vi "Read Manifold Channel Mapping.vi"(8 "error in (no error)":errorcluster, 11 "Gantry in":refnum<class "Gantry.lvclass">) -> (0 "error out":errorcluster, 1 "Port -> Channel":map{i32, i32}(c390), 2 "Channel -> Port":map{i32, i32}(c390), 3 "Gantry out":refnum<class "Gantry.lvclass">)   [LabVIEW 2026, in "Gantry.lvclass"]
uses:
  Gantry.lvclass
  Gantry.lvclass/Gantry.ctl
  FlexWorktable/FlexWorktable.lvclass
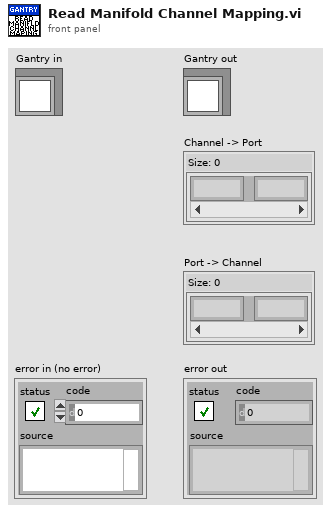
[diagram p1: front panel]
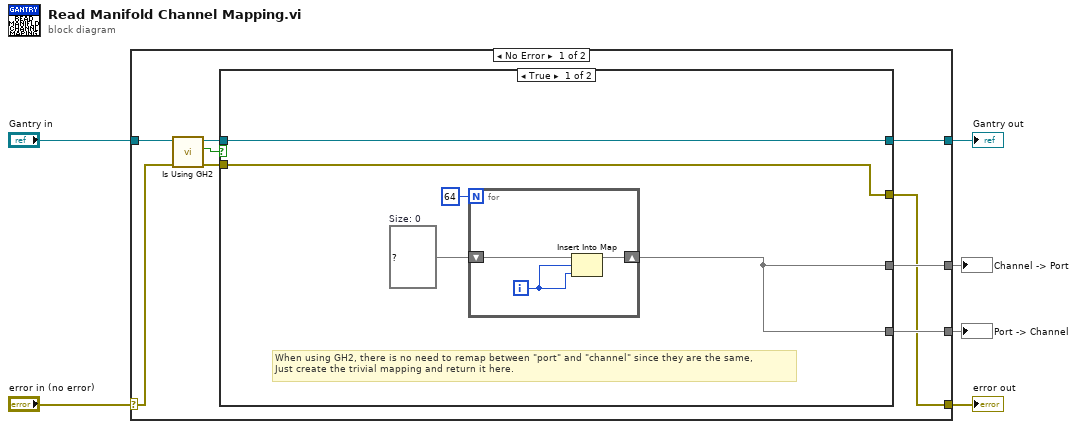
[diagram p0: block diagram]
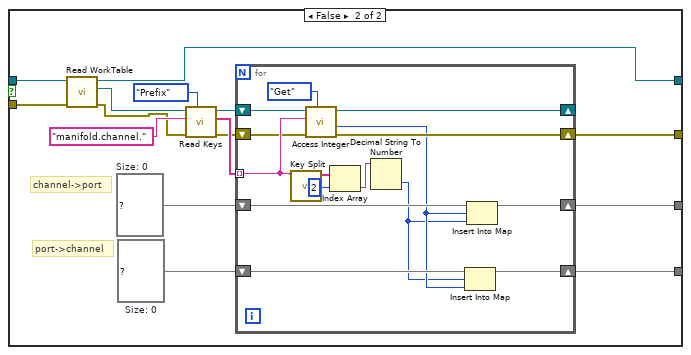
[diagram p2: hidden frame]
diagram:
  n1 = case shown="No Error" "error in (no error)" {
    selector: "error in (no error)" -> [w10 w55]
    tunnel: [w13 w55] -> w5
    tunnel: [w12 w54] -> w3
    tunnel: "Gantry in" -> [w11 w54]
    tunnel: [w15 _] -> w2
    tunnel: [w14 _] -> w1
    frame No Error {
      n2 = call "Is Using GH2.vi"("error in (no error)"=w10, "Gantry in"=w11) -> ("error out"=w9:errorcluster, "Using GH2"=w7:bool, "Gantry out"=w8:refnum<class "Gantry.lvclass">)  [unwired: 7 in]
      n3 = case shown="True" w7 {
        tunnel: w8 -> [w20 w38]
        tunnel: w9 -> [w19 w37]
        tunnel: [w16 w27] -> w15
        tunnel: [w16 w26] -> w14
        tunnel: [w19 w25] -> w13
        tunnel: [w20 w24] -> w12
        frame True {
          w17 = map{i32, i32} {}  # Size: 0
          # "When using GH2, there is no need to remap between \"port\" and \"channel\" since they are the same,\nJust create the trivial mapping and return it here."
          n4 = for {
            N: 64 -> [_]
            shift-right: [w22] -> w16
            shift-left: w17 -> [w23]
            i -> [w21]
            n5 = Insert Into Map(map in=w23, key=w21, value=w21) -> (map out=w22:map{i32, i32})  [unwired: 2 out]
          }
        }
        frame False {
          w30 = map{i32, i32} {}  # Size: 0
          w31 = map{i32, i32} {}  # Size: 0
          # "port->channel"
          # "channel->port"
          n6 = call-dynamic "Read WorkTable.vi"("error in"=w37, "Gantry Class in"=w38) -> ("error out"=w33:errorcluster, "Worktable"=w34:refnum<class "FlexWorktable.lvclass">, "Gantry Class out"=w24:refnum<class "Gantry.lvclass">)  [unwired: 7 in]
          n7 = call-dynamic "Read Keys.vi"("Prefix/Regex"=enum16{"Prefix", "Regex"}."Prefix", "error in (no error)"=w33, "Selector"="manifold.channel.", "FlexWorktable in"=w34) -> ("error out"=w28:errorcluster, "Keys"=w29:string[], "FlexWorktable out"=w32:refnum<class "FlexWorktable.lvclass">)  [unwired: 5 in]
          n8 = for {
            shift-right: [w48] -> _
            shift-left: w32 -> [w49]
            shift-right: [w43] -> w27
            shift-left: w31 -> [w44]
            shift-right: [w41] -> w26
            shift-left: w30 -> [w42]
            tunnel: w29 -> [w53] mode=indexing
            shift-right: [w45] -> w25
            shift-left: w28 -> [w46]
            n9 = call "Key Split.vi"("Key"=w53) -> ("Key Elements"=w52:string[])  [unwired: 10 in]
            n10 = call-dynamic "Access Integer.vi"("Get/Set"=enum16{"Get", "Set"}."Get", "error in (no error)"=w46, "Key"=w53, "FlexWorktable in"=w49) -> ("error out"=w45:errorcluster, "Value out"=w40:i32, "FlexWorktable out"=w48:refnum<class "FlexWorktable.lvclass">)  [unwired: 5 in]
            n11 = Index Array(array=w52, index=2) -> (element=w50:string)
            n12 = Decimal String To Number(string=w50) -> (number=w39:i32)  [unwired: 2 in, 1 out]
            n13 = Insert Into Map(map in=w42, key=w39, value=w40) -> (map out=w41:map{i32, i32})  [unwired: 2 out]
            n14 = Insert Into Map(map in=w44, key=w40, value=w39) -> (map out=w43:map{i32, i32})  [unwired: 2 out]
          }
        }
      }
    }
    frame Error {
    }
  }
  "error out" <- w5
  "Gantry out" <- w3
  "Channel -> Port" <- w2
  "Port -> Channel" <- w1
